vi "Factorize Integer.vi"(1 "Integer in":i32=500) -> (0 "Integer Factors":i32[](array[numeric]))   [LabVIEW 2019, in "Instrument.Lockin.lvlib" / "Instrument.DAQ.lvclass"]
uses:
  Instrument.DAQ.lvclass
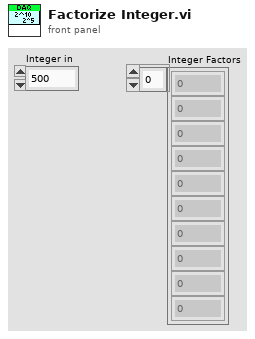
[diagram p1: front panel]
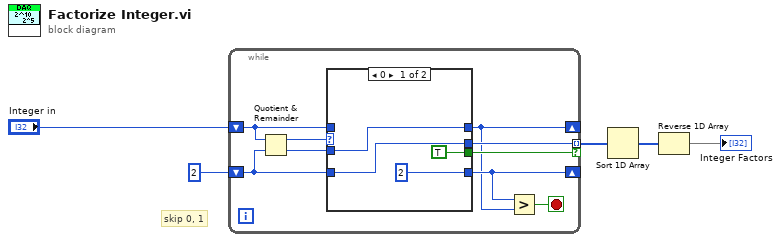
[diagram p0: block diagram]
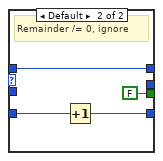
[diagram p2: hidden frame]
diagram:
  # "skip 0, 1"
  n1 = while {
    shift-right: [w7] -> _
    shift-left: "Integer in" -> [w10]
    shift-right: [w8] -> _
    shift-left: 2 -> [w6]
    tunnel: [w12] -> w4 mode=indexing if=w11
    stop <- w9 stop-if-true
    n2 = Quotient & Remainder(x=w10, y=w6) -> (x-y*floor(x/y)=w14:i32, floor(x/y)=w13:i32)
    n3 = case shown="0" w14 {
      tunnel: [w15 w19] -> w7
      tunnel: w13 -> [w15 _]
      tunnel: w6 -> [w16 w22]
      tunnel: [2 w21] -> w8
      tunnel: [w16 _] -> w12
      tunnel: [TRUE FALSE] -> w11
      tunnel: w10 -> [_ w19]
      frame 0 {
      }
      frame Default {
        # "Remainder /= 0, ignore"
        n4 = Increment(x=w22) -> (x+1=w21:i32)
      }
    }
    n5 = Greater?(x=w8, y=w7) -> (0:w9:bool)
  }
  n6 = Sort 1D Array(array=w4) -> (sorted array=w3:i32[])
  n7 = Reverse 1D Array(array=w3) -> (reversed array=→"Integer Factors":i32[])
